vi "TIRF_ReadConfig.vi"(8 "error in (no error)":errorcluster) -> (0 "error out":errorcluster, 1 "Filter Values":T2(array[cluster]), 2 "Laser Values":T3(array[cluster]), 3 "General Settings":T1)   [LabVIEW 2010]
uses:
  <vilib>/Utility/config.llb/Read Key (U32).vi
  <vilib>/Utility/config.llb/Read Key (I32).vi
  <vilib>/Utility/config.llb/Read Key (String).vi
  <vilib>/Utility/config.llb/NI_LVConfig.lvlib
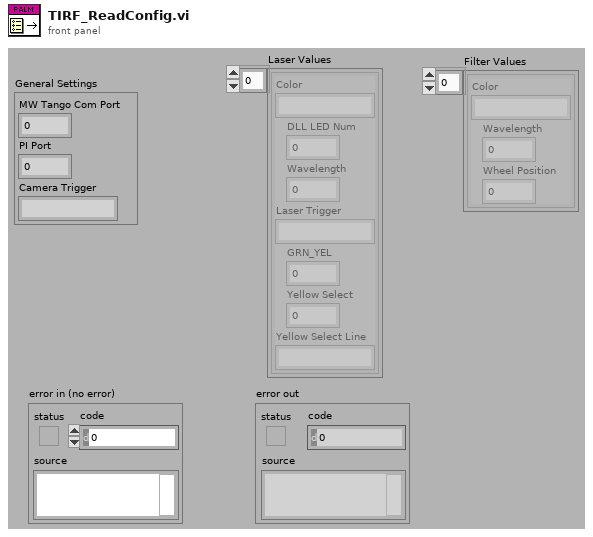
[diagram p1: front panel]
types:
  T1 = cluster{"MW Tango Com Port":u32, "PI Port":i32, "Camera Trigger":string}
  T2 = cluster{"Color":string, "Wavelength":i32, "Wheel Position":i32}[]
  T3 = cluster{"Color":string, "DLL LED Num":i32, "Wavelength":i32, "Laser Trigger":string, "GRN_YEL":i32, "Yellow Select":i32, "Yellow Select Line":string}[]
  T4 = cluster{"Color":string, "Wavelength":i32, "Wheel Position":i32}
  T5 = cluster{"Color":string, "DLL LED Num":i32, "Wavelength":i32, "Counter Name":string, "GRN_YEL":i32, "Yellow Select":i32, "Yellow Select Line":string}
  T6 = typedef "NI_LVConfig.lvlib/Config Data RefNum.ctl" = refnum<k1>
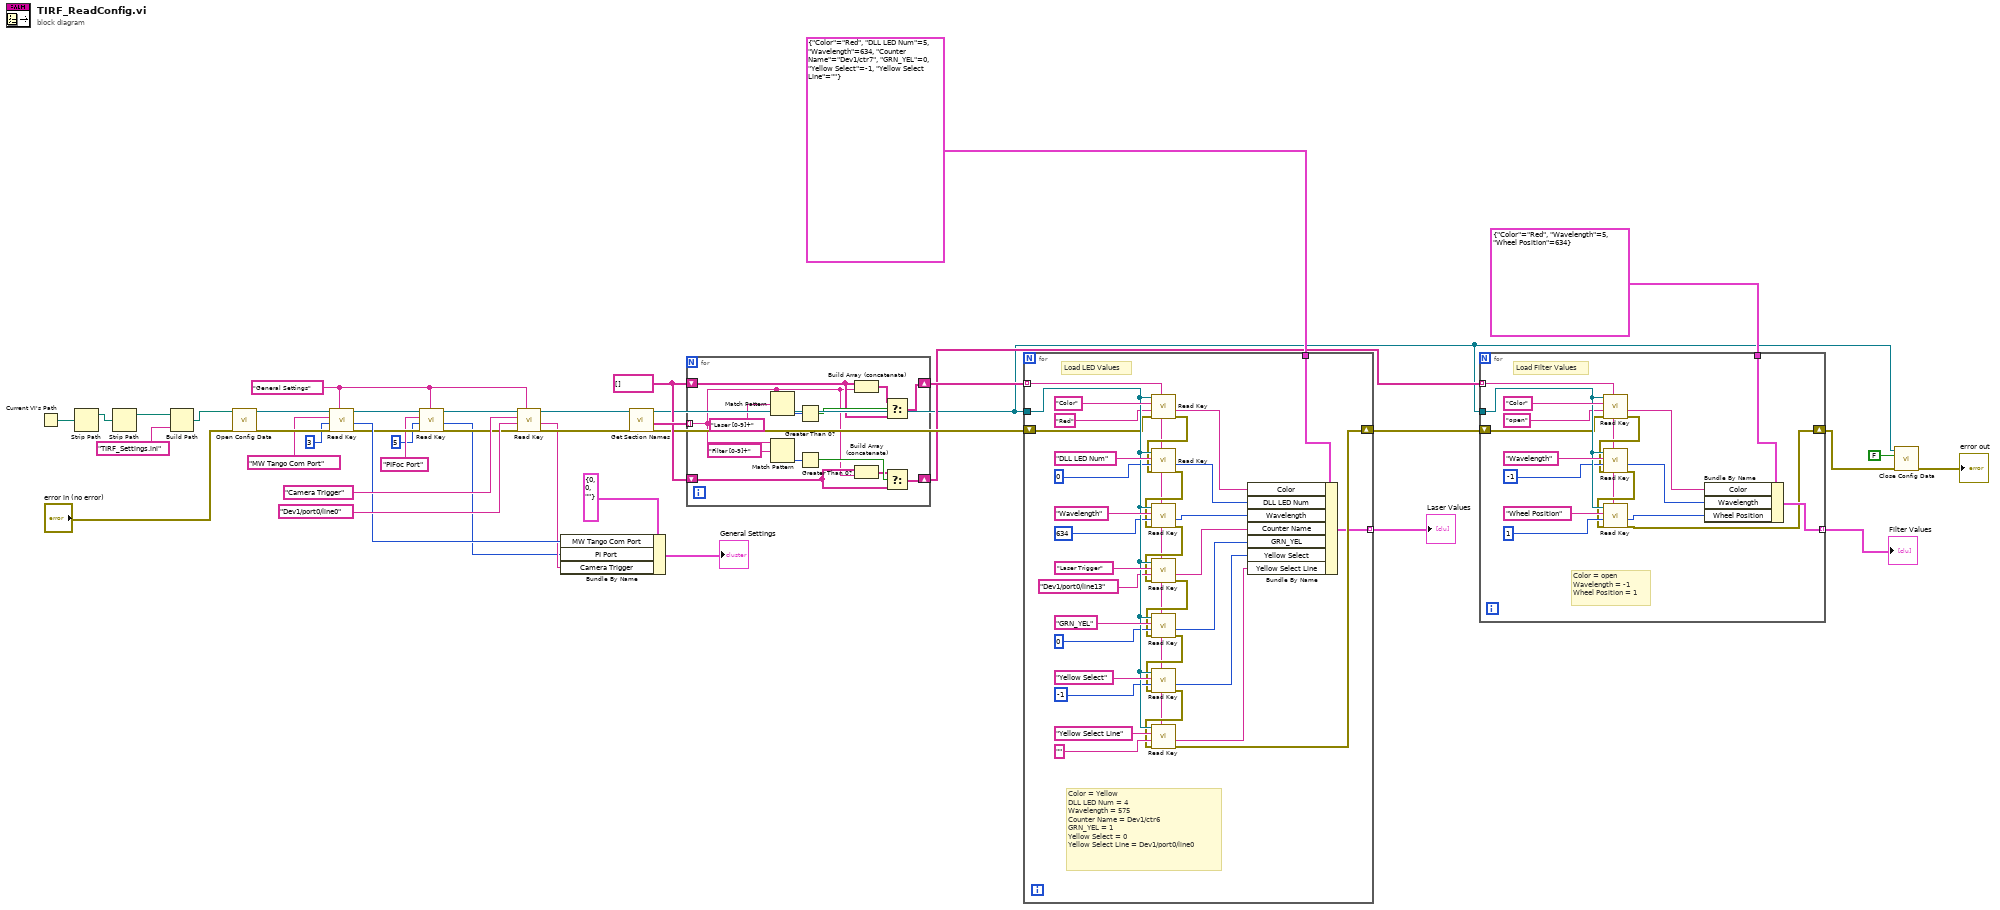
[diagram p0: block diagram]
diagram:
  w31 = string[] []
  w4 = "General Settings" ("section")
  n1 = Current VI's Path() -> (path=w38:path)
  n2 = Strip Path(path=w38) -> (stripped path=w18:path)  [unwired: 1 out]
  n3 = Strip Path(path=w18) -> (stripped path=w17:path)  [unwired: 1 out]
  n4 = Build Path(base path=w17, name or relative path="TIRF_Settings.ini") -> (appended path=w40:path)
  n5 = call <vilib>:"Open Config Data.vi"("error in (no error)"="error in (no error)", "configuration file path"=w40) -> ("error out"=w36:errorcluster, "refnum"=w35:T6)  [unwired: 7 in, 1 out]
  n6 = call-poly <vilib>:"Read Key.vi"("section"=w4, "error in (no error)"=w36, "default value"=u32 3, "key"="MW Tango Com Port" ("section"), "refnum"=w35) -> ("error out"=w8:errorcluster, "value"=w12:u32, "refnum out"=w6:T6)  [unwired: 3 in, 1 out]
  n7 = call-poly <vilib>:"Read Key.vi"("section"=w4, "error in (no error)"=w8, "default value"=5, "key"="PIFoc Port" ("section"), "refnum"=w6) -> ("error out"=w7:errorcluster, "value"=w1:i32, "refnum out"=w5:T6)  [unwired: 3 in, 1 out]
  n8 = call-poly <vilib>:"Read Key.vi"("section"=w4, "error in (no error)"=w7, "default value"="Dev1/port0/line0" ("section"), "key"="Camera Trigger" ("section"), "refnum"=w5) -> ("error out"=w16:errorcluster, "value"=w9:string, "refnum out"=w13:T6)  [unwired: 3 in, 1 out]
  n9 = Bundle By Name(cluster=T1 {"MW Tango Com Port"=0, "PI Port"=0, "Camera Trigger"=""} ("General Settings"), "MW Tango Com Port"=w12, "PI Port"=w1, "Camera Trigger"=w9) -> (→"General Settings":T1)
  n10 = call <vilib>:"Get Section Names.vi"("error in (no error)"=w16, "refnum"=w13) -> ("error out"=w29:errorcluster, "section names"=w32:string[], "refnum out"=w23:T6)  [unwired: 7 in]
  n11 = for {
    tunnel: w32 -> [w42] mode=indexing
    shift-right: [w47] -> w30
    shift-left: w31 -> [w43]
    shift-right: [w41] -> w25
    shift-left: w31 -> [w44]
    n12 = Match Pattern(string=w42, regular expression="Laser [0-9]+") -> (offset past match=w50:i32)  [unwired: 1 in, 3 out]
    n13 = Match Pattern(string=w42, regular expression="Filter [0-9]+") -> (offset past match=w51:i32)  [unwired: 1 in, 3 out]
    n14 = Greater Than 0?(x=w50) -> (x > 0?=w49:bool)
    n15 = Greater Than 0?(x=w51) -> (x > 0?=w48:bool)
    n16 = Build Array (concatenate)(w43, w42) -> (w46:string[])
    n17 = Build Array (concatenate)(w44, w42) -> (w45:string[])
    n18 = Select(t=w46, s=w49, f=w43) -> (s? t:f=w47:string[])
    n19 = Select(t=w45, s=w48, f=w44) -> (s? t:f=w41:string[])
  }
  n20 = for {
    tunnel: w30 -> [w63] mode=indexing
    shift-right: [w64] -> w26
    shift-left: w29 -> [w72]
    tunnel: w23 -> [w79]
    tunnel: T5 {"Color"="Red", "DLL LED Num"=5, "Wavelength"=634, "Counter Name"="Dev1/ctr7", "GRN_YEL"=0, "Yellow Select"=-1, "Yellow Select Line"=""} -> [w62]
    tunnel: [w54] -> w27 mode=indexing
    # "Color = Yellow\nDLL LED Num = 4\nWavelength = 575\nCounter Name = Dev1/ctr6\nGRN_YEL = 1\nYellow Select = 0\nYellow Select Line = Dev1/port0/line0"
    # "Load LED Values"
    n21 = call-poly <vilib>:"Read Key.vi"("section"=w63, "error in (no error)"=w72, "default value"="Red", "key"="Color", "refnum"=w79) -> ("error out"=w71:errorcluster, "value"=w61:string)  [unwired: 3 in, 2 out]
    n22 = call-poly <vilib>:"Read Key.vi"("section"=w63, "error in (no error)"=w71, "default value"=0, "key"="DLL LED Num", "refnum"=w79) -> ("error out"=w70:errorcluster, "value"=w60:i32)  [unwired: 3 in, 2 out]
    n23 = call-poly <vilib>:"Read Key.vi"("section"=w63, "error in (no error)"=w70, "default value"=634, "key"="Wavelength", "refnum"=w79) -> ("error out"=w69:errorcluster, "value"=w59:i32)  [unwired: 3 in, 2 out]
    n24 = call-poly <vilib>:"Read Key.vi"("section"=w63, "error in (no error)"=w69, "default value"="Dev1/port0/line13", "key"="Laser Trigger", "refnum"=w79) -> ("error out"=w67:errorcluster, "value"=w55:string)  [unwired: 3 in, 2 out]
    n25 = call-poly <vilib>:"Read Key.vi"("section"=w63, "error in (no error)"=w67, "default value"=0, "key"="GRN_YEL", "refnum"=w79) -> ("error out"=w66:errorcluster, "value"=w57:i32)  [unwired: 3 in, 2 out]
    n26 = call-poly <vilib>:"Read Key.vi"("section"=w63, "error in (no error)"=w66, "default value"=-1, "key"="Yellow Select", "refnum"=w79) -> ("error out"=w65:errorcluster, "value"=w56:i32)  [unwired: 3 in, 2 out]
    n27 = call-poly <vilib>:"Read Key.vi"("section"=w63, "error in (no error)"=w65, "default value"="", "key"="Yellow Select Line", "refnum"=w79) -> ("error out"=w64:errorcluster, "value"=w58:string)  [unwired: 3 in, 2 out]
    n28 = Bundle By Name(cluster=w62, "Color"=w61, "DLL LED Num"=w60, "Wavelength"=w59, "Counter Name"=w55, "GRN_YEL"=w57, "Yellow Select"=w56, "Yellow Select Line"=w58) -> (w54:T5)
  }
  "Laser Values" <- w27
  n29 = for {
    tunnel: w25 -> [w93] mode=indexing
    shift-right: [w87] -> w21
    shift-left: w26 -> [w96]
    tunnel: w23 -> [w100]
    tunnel: T4 {"Color"="Red", "Wavelength"=5, "Wheel Position"=634} -> [w92]
    tunnel: [w88] -> w19 mode=indexing
    # "Color = open\nWavelength = -1\nWheel Position = 1"
    # "Load Filter Values"
    n30 = call-poly <vilib>:"Read Key.vi"("section"=w93, "error in (no error)"=w96, "default value"="open", "key"="Color", "refnum"=w100) -> ("error out"=w95:errorcluster, "value"=w91:string)  [unwired: 3 in, 2 out]
    n31 = call-poly <vilib>:"Read Key.vi"("section"=w93, "error in (no error)"=w95, "default value"=-1, "key"="Wavelength", "refnum"=w100) -> ("error out"=w94:errorcluster, "value"=w90:i32)  [unwired: 3 in, 2 out]
    n32 = call-poly <vilib>:"Read Key.vi"("section"=w93, "error in (no error)"=w94, "default value"=1, "key"="Wheel Position", "refnum"=w100) -> ("error out"=w87:errorcluster, "value"=w89:i32)  [unwired: 3 in, 2 out]
    n33 = Bundle By Name(cluster=w92, "Color"=w91, "Wavelength"=w90, "Wheel Position"=w89) -> (w88:T4)
  }
  "Filter Values" <- w19
  n34 = call <vilib>:"Close Config Data.vi"("error in (no error)"=w21, "write file if changed (T)"=FALSE, "refnum"=w23) -> ("error out"=→"error out":errorcluster)  [unwired: 7 in, 1 out]
